vi "format into Sonde Vertical Graph Data Input.vi"(9 "Sonde Measurement Array":dbl[][](array[numeric]), 11 "Time Array":dbl[](array[numeric])) -> (2 "Sonde Data Display":T1, 5 "Temperature":cluster{"X":dbl[], "Y":dbl[]}[](array[cluster]))   [LabVIEW 2016]
uses:
  SDI-12/Sonde Vertical Graph.ctl
  controls/Vertical Chart.ctl
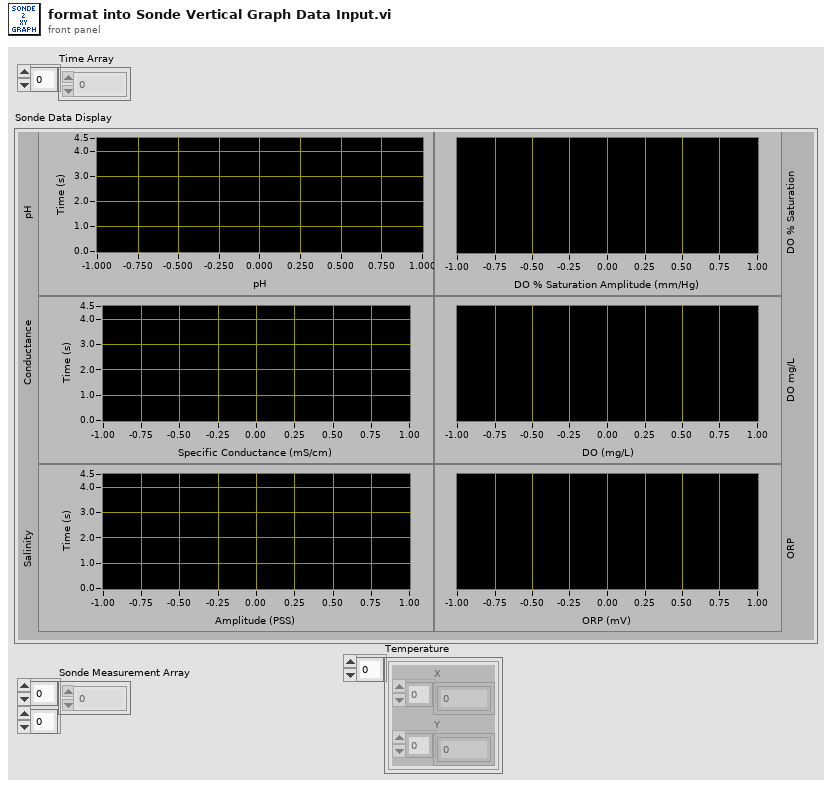
[diagram p1: front panel]
types:
  T1 = typedef "Sonde Vertical Graph.ctl" = cluster{"pH":T2, "Conductance":T2, "Salinity":T2, "DO % Saturation":T2, "DO mg/L":T2, "ORP":T2}
  T2 = typedef "Vertical Chart.ctl" = cluster{"Y":dbl[], "Y":dbl[]}[]
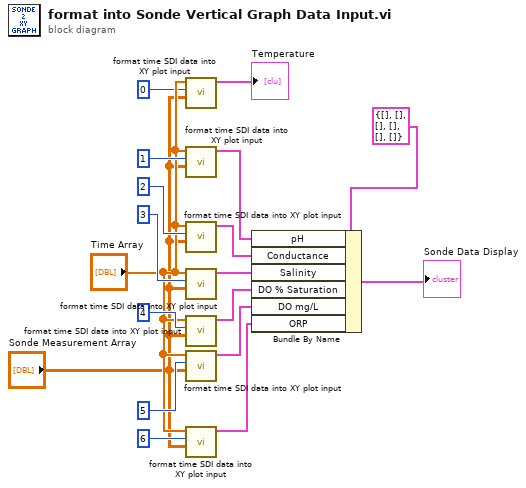
[diagram p0: block diagram]
diagram:
  n1 = call "format time SDI data into XY plot input.vi"("Measurement Array"="Sonde Measurement Array", "disabled index (col)"=0, "Time Array"="Time Array") -> ("XY Graph"=→"Temperature":cluster{"X":dbl[], "Y":dbl[]}[])  [unwired: 8 in]
  n2 = call "format time SDI data into XY plot input.vi"("Measurement Array"="Sonde Measurement Array", "disabled index (col)"=1, "Time Array"="Time Array") -> ("XY Graph"=w11:cluster{"X":dbl[], "Y":dbl[]}[])  [unwired: 8 in]
  n3 = call "format time SDI data into XY plot input.vi"("Measurement Array"="Sonde Measurement Array", "disabled index (col)"=2, "Time Array"="Time Array") -> ("XY Graph"=w12:cluster{"X":dbl[], "Y":dbl[]}[])  [unwired: 8 in]
  n4 = call "format time SDI data into XY plot input.vi"("Measurement Array"="Sonde Measurement Array", "disabled index (col)"=3, "Time Array"="Time Array") -> ("XY Graph"=w13:cluster{"X":dbl[], "Y":dbl[]}[])  [unwired: 8 in]
  n5 = call "format time SDI data into XY plot input.vi"("Measurement Array"="Sonde Measurement Array", "disabled index (col)"=4, "Time Array"="Time Array") -> ("XY Graph"=w14:cluster{"X":dbl[], "Y":dbl[]}[])  [unwired: 8 in]
  n6 = call "format time SDI data into XY plot input.vi"("Measurement Array"="Sonde Measurement Array", "disabled index (col)"=5, "Time Array"="Time Array") -> ("XY Graph"=w9:cluster{"X":dbl[], "Y":dbl[]}[])  [unwired: 8 in]
  n7 = call "format time SDI data into XY plot input.vi"("Measurement Array"="Sonde Measurement Array", "disabled index (col)"=6, "Time Array"="Time Array") -> ("XY Graph"=w7:cluster{"X":dbl[], "Y":dbl[]}[])  [unwired: 8 in]
  n8 = Bundle By Name(cluster=T1 {"pH"=[], "Conductance"=[], "Salinity"=[], "DO % Saturation"=[], "DO mg/L"=[], "ORP"=[]} ("Sonde Data Display"), "pH"=w11, "Conductance"=w12, "Salinity"=w13, "DO % Saturation"=w14, "DO mg/L"=w9, "ORP"=w7) -> (→"Sonde Data Display":T1)
